vi "HB_ReadAI.vi"   [LabVIEW 2018]
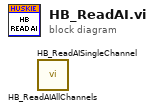
[diagram p0: block diagram]
diagram:
  n1 = call "HB_ReadAIAllChannels.vi"() -> ()  [unwired: 8 in, 4 out]
  n2 = call "HB_ReadAISingleChannel.vi"() -> ()  [unwired: 8 in, 4 out]
